vi "ExecuteMenuCommand.vi"(0 "reference":refnum<class "AbstractNode.lvclass">, 1 "Command":string, 5 "error in (no error)":errorcluster) -> (14 "reference out":refnum<class "AbstractNode.lvclass">, 15 "EditorAction":T3, 16 "FlattenCommandSettings":T1, 19 "error out":errorcluster)   [LabVIEW 2014, in "AbstractNode.lvclass"]
uses:
  <resource>/Framework/Providers/Open_GDS/UML/AbstractNode_class/AbstractNode.lvclass
  <resource>/Framework/Providers/Open_GDS/UML/UMLEditor/UMLEditor EditorActionType.ctl
  <resource>/Framework/Providers/Open_GDS/UML/UMLEditor/UMLEditor FlattenCommandType.ctl
  <resource>/Framework/Providers/Open_GDS/UML/UMLEditor/UMLEditor ExecuteCommandType.ctl
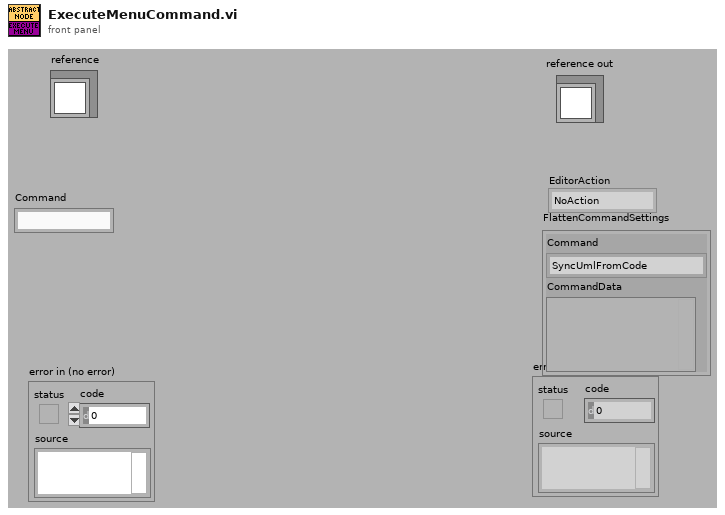
[diagram p1: front panel]
types:
  T1 = typedef "UMLEditor FlattenCommandType.ctl" = cluster{"Command":T2, "CommandData":variant}
  T2 = typedef "UMLEditor ExecuteCommandType.ctl" = enum16{"SyncUmlFromCode", "SyncCodeFromUML", "OpenClass", "OpenFile", "CreateClass", "CreateVI", "OpenClassAttribute", "LocateInProject"}
  T3 = typedef "UMLEditor EditorActionType.ctl" = enum16{"NoAction", "Repaint", "ExecuteCommand"}
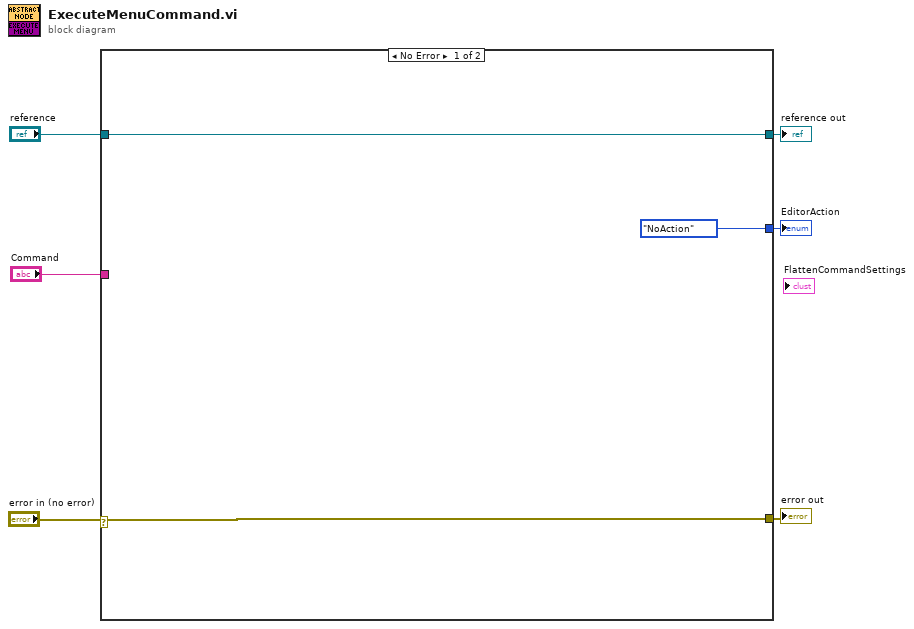
[diagram p0: block diagram]
diagram:
  n1 = case shown="No Error" "error in (no error)" {
    selector: "error in (no error)" -> [w8 w10]
    tunnel: "reference" -> [w9 w11]
    tunnel: [w8 w10] -> w5
    tunnel: [w9 w11] -> w4
    tunnel: "Command" -> [_ _]
    tunnel: [UMLEditor_EditorActionType."NoAction" ("EditorAction") _] -> w1
    frame No Error {
    }
    frame Error {
    }
  }
  "reference out" <- w4
  "error out" <- w5
  "EditorAction" <- w1
